vi "Mutate_v1_to_v2.vi"(11 "SerializableData_v1":T2) -> (0 "error out":errorcluster, 3 "SerializableData":T1)   [LabVIEW 2019, in "Golf Club.lvclass"]
uses:
  Golf Club.lvclass
  SerializableData_v1.ctl
  SerializableData.ctl
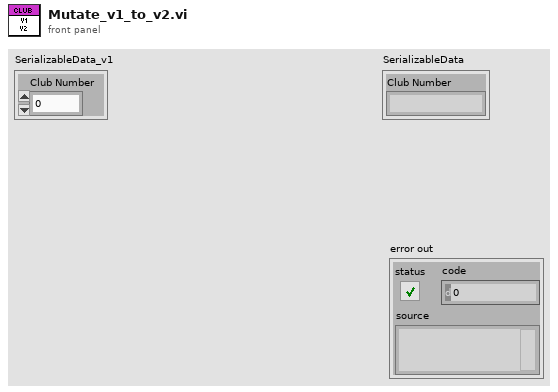
[diagram p1: front panel]
types:
  T1 = typedef "Golf Club.lvclass/SerializableData.ctl" = cluster{"Club Number":string}
  T2 = typedef "Golf Club.lvclass/SerializableData_v1.ctl" = cluster{"Club Number":i32}
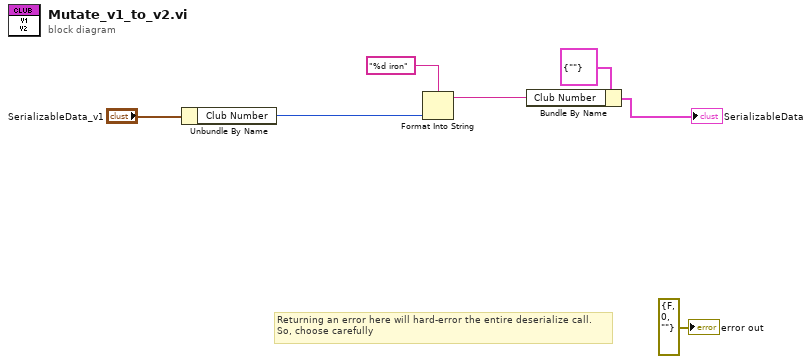
[diagram p0: block diagram]
diagram:
  # "Returning an error here will hard-error the entire deserialize call.\nSo, choose carefully"
  n1 = Unbundle By Name("SerializableData_v1") -> ("Club Number"=w5:i32)
  n2 = Format Into String(format string="%d iron", w5) -> (resulting string=w2:string)  [unwired: 2 in, 1 out]
  n3 = Bundle By Name(cluster=T1 {"Club Number"=""} ("SerializableData"), "Club Number"=w2) -> (→"SerializableData":T1)
  "error out" <- errorcluster {"status"=FALSE, "code"=0, "source"=""} ("error out")
